vi "Unit Discrete Delay (U32).vi"(7 "Input":u32) -> (8 "Output":u32)   [LabVIEW 2011]
uses:
  <vilib>/rvi/FXPMathLib/basic elements/FxpDiscreteDelay/XNode/nifxpmath_DiscreteDelay.xnode
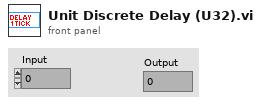
[diagram p1: front panel]
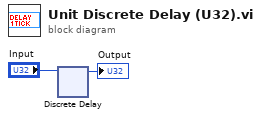
[diagram p0: block diagram]
diagram:
  n1 = xnode "Discrete Delay"("D"="Input") -> ("Q"=→"Output":u32)
